vi "Display Info.vi"(7 "Layout ref":refnum<vi>, 8 "error in (no error)":errorcluster, 9 "Modify (F) /Add [T]":bool, 10 "Names in use":string[](array[string]), 11 "Advanced_DMD in":refnum<class "Advanced_DMD.lvclass">) -> (0 "error out":errorcluster, 1 "Names in use out":string[](array[string]), 2 "Changes Made?":bool, 3 "Advanced_DMD out":refnum<class "Advanced_DMD.lvclass">)   [LabVIEW 2013, in "Advanced_DMD.lvclass"]
uses:
  Advanced_DMD.lvclass
  TypeDefs/ColumnAppearCluster.ctl
  Advanced_DMD.lvclass/Advanced_DMD.ctl
  ColumnVIs/Column/Column.lvclass
panel:
  in  "Mode Appearance":T1={"Column Name"="Num Images", "Width"=30, "Bkgd"=[16448250], "Text"=[0]}
  in  "Image Cluster":T2
  in  "Argument Column Appearance":T1={"Column Name"="Column_0", "Width"=30, "Bkgd"=[16448250], "Text"=[0]}
  in  "Program Mode Appearance":T1={"Column Name"="Program Mode", "Width"=30, "Bkgd"=[16448250], "Text"=[0]}
  in  "Display Mode Appearance":T1={"Column Name"="Disp Mode", "Width"=30, "Bkgd"=[16448250], "Text"=[0]}
  in  "Device Description":string
  in  "Hardware Settings":T3={"IP Address"="172.16.1.100", "Image Root Path"=path "C:/Users/Lab/Google Drive/Sr/ToOrganize/Strontium Experiment/DLP3000 codes/Matlab codes/Sr_Matlab", "Port"=21845} {"Port" format="%x"}
  in  "Name":string
  in  "Done":bool
  in  "Cancel":bool
  # "Use IP addresses in: \n172.16.0.0 to 172.16.255.255\nor\n192.168.0.0 to 192.168.255.255\ncurrent setting: 172.16.1.100\n\nNote: Most DMDs default to\n192.168.1.100\n\nIf another IP is needed it must be \nset with the DMD software."
  # "This VI just sets the wiring structure.\nOpen a child override version instead!"
  # "Always use Port 0x5555\nPort Field is in Hexadecimal"
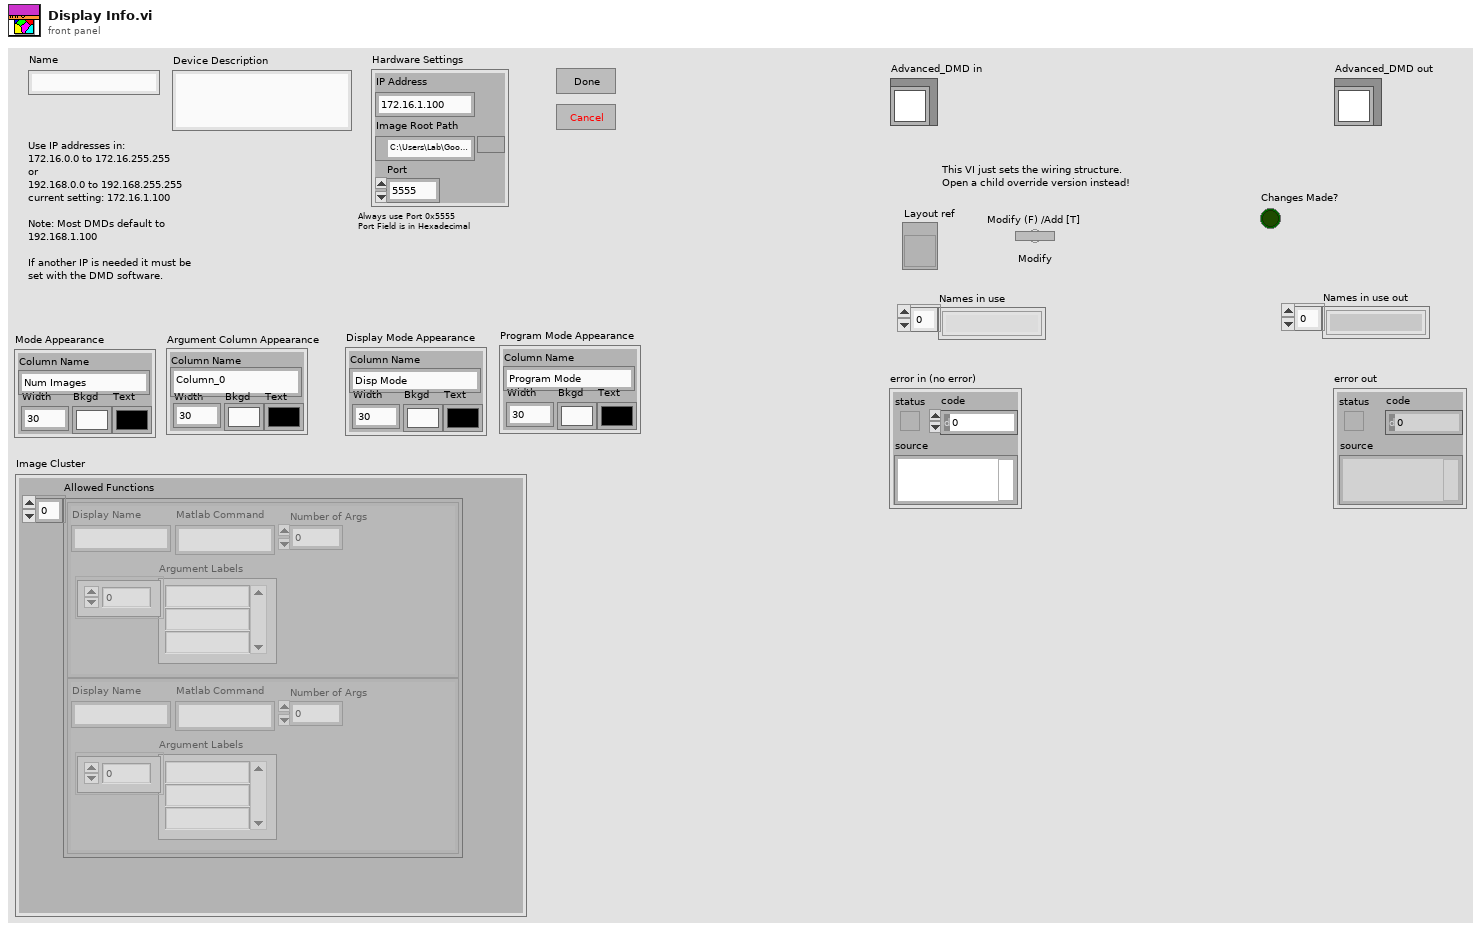
[diagram p1: front panel]
types:
  T1 = typedef "ColumnAppearCluster.ctl" = cluster{"Column Name":string, "Width":u32, "Bkgd":u32[], "Text":u32[]}
  T2 = cluster{"Allowed Functions":cluster{"Display Name":string, "Matlab Command":string, "Number of Args":u8, "Argument Labels":string[]}[]}
  T3 = cluster{"IP Address":string, "Image Root Path":path, "Port":u16}
  T4 = cluster{"Display Name":string, "Matlab Command":string, "Number of Args":u8, "Argument Labels":string[]}[]
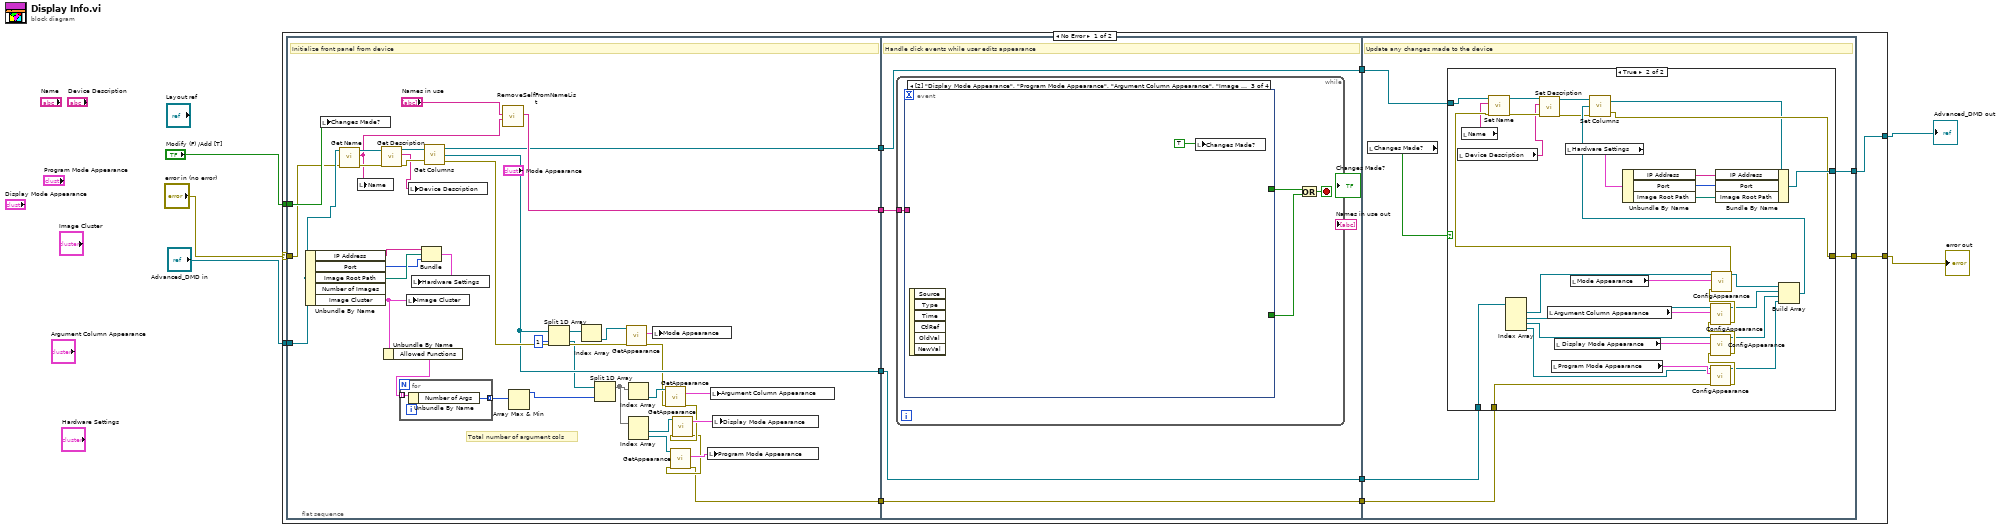
[diagram p0: block diagram]
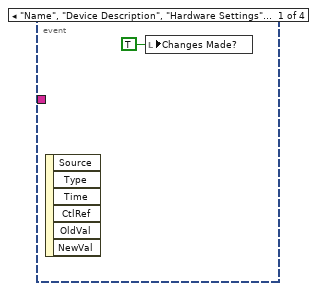
[diagram p2: hidden frame]
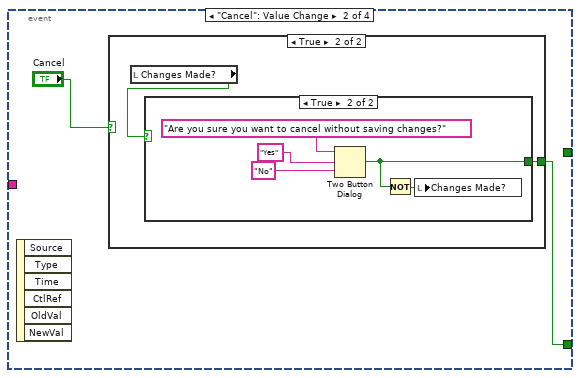
[diagram p3: hidden frame]
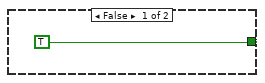
[diagram p5: hidden frame]
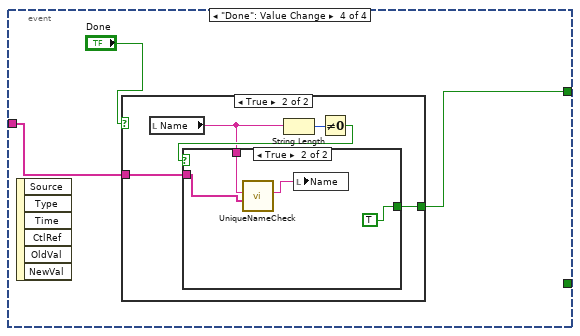
[diagram p6: hidden frame]
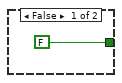
[diagram p7: hidden frame]
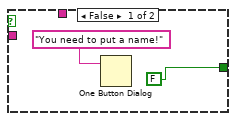
[diagram p8: hidden frame]
diagram:
  n1 = case shown="No Error" "error in (no error)" {
    selector: "error in (no error)" -> [w15 w136]
    tunnel: [w7 w136] -> w1
    tunnel: [w6 w135] -> w2
    tunnel: "Advanced_DMD in" -> [w16 w135]
    tunnel: "Modify (F) /Add [T]" -> [w17 _]
    frame No Error {
      n2 = flat-sequence {
        tunnel: w17 -> [w55]
        tunnel: w16 -> [w53]
        tunnel: w15 -> [w51]
        tunnel: [w43] -> w14
        tunnel: [w42] -> w13
        tunnel: [w35] -> w11
        tunnel: [w19] -> w9
        tunnel: w14 -> [w61]
        tunnel: w13 -> [w60]
        tunnel: [w60] -> w12
        tunnel: w11 -> [w59]
        tunnel: [w59] -> w10
        tunnel: w9 -> [w58]
        tunnel: [w58] -> w8
        tunnel: w12 -> [w99]
        tunnel: w10 -> [w98]
        tunnel: w8 -> [w97]
        tunnel: [w95] -> w7
        tunnel: [w94] -> w6
        frame #0 {
          # "Total number of argument cols"
          # "Initialize front panel from device"
          n3 = Unbundle By Name(w53) -> ("IP Address"=w54:string, "Port"=w40:u16, "Image Root Path"=w41:path, "Image Cluster"=w18:T2)  [unwired: 1 out]
          n4 = local write "Changes Made?"(w55) -> ()
          n5 = call-dynamic "Get Name.vi"("error in (no error)"=w51, "Device in"=w53) -> ("error out"=w50:errorcluster, "Name"=w47:string, "Device out"=w52:refnum<class "Advanced_DMD.lvclass">)  [unwired: 7 in]
          n6 = local write "Name"(w47) -> ()
          n7 = call-dynamic "Get Description.vi"("error in (no error)"=w50, "Device in"=w52) -> ("error out"=w48:errorcluster, "Device Description"=w46:string, "Device out"=w49:refnum<class "Advanced_DMD.lvclass">)  [unwired: 7 in]
          n8 = Unbundle By Name(w18) -> ("Allowed Functions"=w37:T4)
          n9 = for {
            tunnel: w37 -> [w57] mode=indexing
            tunnel: [w56] -> w36 mode=indexing
            n10 = Unbundle By Name(w57) -> ("Number of Args"=w56:u8)
          }
          n11 = local write "Image Cluster"(w18) -> ()
          n12 = local write "Device Description"(w46) -> ()
          n13 = Bundle("IP Address"=w54, "Image Root Path"=w41, "Port"=w40) -> (w39:T3)  [unwired: 1 in]
          n14 = local write "Hardware Settings"(w39) -> ()
          n15 = call-dynamic "Get Columns.vi"("Device in"=w49, "error in (no error)"=w48) -> ("Device out"=w42:refnum<class "Advanced_DMD.lvclass">, "Columns"=w35:refnum<class "Column.lvclass">[], "error out"=w45:errorcluster)
          n16 = call "RemoveSelfFromNameList.vi"("self Name"=w47, "Names in use"="Names in use") -> ("Reserved Names"=w43:string[])  [unwired: 9 in]
          n17 = Array Max & Min(array=w36) -> (max value=w31:u8)  [unwired: 3 out]
          n18 = Split 1D Array(array=w35, index=1) -> (first subarray=w33:refnum<class "Column.lvclass">[], second subarray=w30:refnum<class "Column.lvclass">[])
          n19 = Index Array(array=w33) -> (element=w32:refnum<class "Column.lvclass">)  [unwired: 1 in]
          n20 = Split 1D Array(array=w30, index=w31) -> (first subarray=w27:refnum<class "Column.lvclass">[])  [unwired: 1 out]
          n21 = call "GetAppearance.vi"("error in (no error)"=w45, "Column in"=w32) -> ("error out"=w22:errorcluster, "Column Appearance"=w44:T1)  [unwired: 7 in, 1 out]
          n22 = Index Array(array=w27) -> (element=w29:refnum<class "Column.lvclass">)  [unwired: 1 in]
          n23 = Index Array(array=w27) -> (element #1=w26:refnum<class "Column.lvclass">, element #2=w25:refnum<class "Column.lvclass">)  [unwired: 2 in]
          n24 = local write "Mode Appearance"(w44) -> ()
          n25 = call "GetAppearance.vi"("error in (no error)"=w22, "Column in"=w29) -> ("error out"=w21:errorcluster, "Column Appearance"=w28:T1)  [unwired: 7 in, 1 out]
          n26 = call "GetAppearance.vi"("error in (no error)"=w21, "Column in"=w26) -> ("error out"=w20:errorcluster, "Column Appearance"=w24:T1)  [unwired: 7 in, 1 out]
          n27 = call "GetAppearance.vi"("error in (no error)"=w20, "Column in"=w25) -> ("error out"=w19:errorcluster, "Column Appearance"=w23:T1)  [unwired: 7 in, 1 out]
          n28 = local write "Program Mode Appearance"(w23) -> ()
          n29 = local write "Argument Column Appearance"(w28) -> ()
          n30 = local write "Display Mode Appearance"(w24) -> ()
        }
        frame #1 {
          # "Handle click events while user edits appearance"
          n31 = while {
            tunnel: w61 -> [w62]
            stop <- w65 stop-if-true
            n32 = event shown="[2] \"Display Mode Appearance\", \"Program Mode Appearance\", \"Argument Column Appearance\", \"Image Cluster\", \"Mode Appearance\": Value Change" {
              selector: _ -> [_ _ _ _]
              dyn-events: _ -> [_ _ _ _]
              timeout: _ -> [_ _ _ _]
              tunnel: [_ w68 _ _] -> w64
              tunnel: [_ _ _ w81] -> w63
              tunnel: w62 -> [_ _ _ w80]
              event "Name", "Device Description", "Hardware Settings": Value Change {
                n33 = event-data() -> ()  [unwired: 1 in, 6 out]
                n34 = local write "Changes Made?"(TRUE ("Changes Made?")) -> ()
              }
              event "Cancel": Value Change {
                n35 = event-data() -> ()  [unwired: 1 in, 6 out]
                n36 = case shown="True" "Cancel" {
                  selector: "Cancel" -> [w69 _]
                  tunnel: [w69 w71] -> w68
                  frame False {
                  }
                  frame True {
                    n37 = local read "Changes Made?"() -> (w70:bool)
                    n38 = case shown="True" w70 {
                      tunnel: [TRUE w74] -> w71
                      frame False {
                      }
                      frame True {
                        n39 = Two Button Dialog(message="Are you sure you want to cancel without saving changes?", 1:"No", 2:"Yes") -> (T button?=w74:bool)
                        n40 = Not(x=w74) -> (.not. x?=w73:bool)
                        n41 = local write "Changes Made?"(w73) -> ()
                      }
                    }
                  }
                }
              }
              event "Image Cluster": Value Change {
                n42 = event-data() -> ()  [unwired: 1 in, 6 out]
                n43 = local write "Changes Made?"(TRUE) -> ()
              }
              event "Done": Value Change {
                n44 = event-data() -> ()  [unwired: 1 in, 6 out]
                n45 = case shown="True" "Done" {
                  tunnel: [FALSE w85] -> w81
                  tunnel: w80 -> [_ w84]
                  frame False {
                  }
                  frame True {
                    n46 = local read "Name"() -> (w83:string)
                    n47 = String Length(string=w83) -> (length=w87:i32)
                    n48 = Not Equal To 0?(x=w87) -> (x != 0?=w86:bool)
                    n49 = case shown="True" w86 {
                      tunnel: [FALSE TRUE] -> w85
                      tunnel: w84 -> [_ w92]
                      tunnel: w83 -> [_ w91]
                      frame False {
                        n50 = One Button Dialog(message="You need to put a name!") -> ()  [unwired: 1 in, 1 out]
                      }
                      frame True {
                        n51 = call "UniqueNameCheck.vi"("Names in use"=w92, "Device Name"=w91) -> ("Unique name"=w90:string)  [unwired: 8 in, 1 out]
                        n52 = local write "Name"(w90) -> ()
                      }
                    }
                  }
                }
              }
            }
            n53 = Or(x=w63, y=w64) -> (x .or. y?=w65:bool)
          }
        }
        frame #2 {
          # "Update any changes made to the device"
          n54 = local read "Changes Made?"() -> (w96:bool)
          n55 = case shown="True" w96 {
            tunnel: w99 -> [w101 w134]
            tunnel: w98 -> [_ w132]
            tunnel: w97 -> [w100 w109]
            tunnel: [w100 w111] -> w95
            tunnel: [w101 w114] -> w94
            frame False {
            }
            frame True {
              n56 = local read "Device Description"() -> (w102:string)
              n57 = local read "Name"() -> (w103:string)
              n58 = Index Array(array=w132) -> (element #1=w131:refnum<class "Column.lvclass">, element #2=w130:refnum<class "Column.lvclass">, element #3=w129:refnum<class "Column.lvclass">, element #4=w106:refnum<class "Column.lvclass">)  [unwired: 4 in]
              n59 = local read "Argument Column Appearance"() -> (w123:T1)
              n60 = local read "Program Mode Appearance"() -> (w107:T1)
              n61 = local read "Display Mode Appearance"() -> (w122:T1)
              n62 = local read "Hardware Settings"() -> (w104:T3)
              n63 = local read "Mode Appearance"() -> (w124:T1)
              n64 = Unbundle By Name(w104) -> ("IP Address"=w115:string, "Port"=w113:u16, "Image Root Path"=w112:path)
              n65 = call "ConfigAppearance.vi"("error in (no error)"=w109, "Column Appearance"=w107, "Column in"=w106) -> ("error out"=w108:errorcluster, "Column out"=w105:refnum<class "Column.lvclass">)  [unwired: 7 in]
              n66 = call "ConfigAppearance.vi"("error in (no error)"=w108, "Column Appearance"=w122, "Column in"=w129) -> ("error out"=w128:errorcluster, "Column out"=w119:refnum<class "Column.lvclass">)  [unwired: 7 in]
              n67 = call "ConfigAppearance.vi"("error in (no error)"=w128, "Column Appearance"=w123, "Column in"=w130) -> ("error out"=w127:errorcluster, "Column out"=w120:refnum<class "Column.lvclass">)  [unwired: 7 in]
              n68 = call "ConfigAppearance.vi"("error in (no error)"=w127, "Column Appearance"=w124, "Column in"=w131) -> ("error out"=w126:errorcluster, "Column out"=w121:refnum<class "Column.lvclass">)  [unwired: 7 in]
              n69 = call-dynamic "Set Name.vi"("error in (no error)"=w126, "Name"=w103, "Device in"=w134) -> ("error out"=w125:errorcluster, "Device out"=w133:refnum<class "Advanced_DMD.lvclass">)  [unwired: 7 in]
              n70 = call-dynamic "Set Description.vi"("error in (no error)"=w125, "Device Description"=w102, "Device in"=w133) -> ("error out"=w116:errorcluster, "Device out"=w117:refnum<class "Advanced_DMD.lvclass">)  [unwired: 7 in]
              n71 = Build Array(w121, w120, w119, w105) -> (w118:refnum<class "Column.lvclass">[])
              n72 = call-dynamic "Set Columns.vi"("error in (no error)"=w116, "Columns"=w118, "Device in"=w117) -> ("error out"=w111:errorcluster, "Device out"=w110:refnum<class "Advanced_DMD.lvclass">)  [unwired: 1 in]
              n73 = Bundle By Name(cluster=w110, "IP Address"=w115, "Port"=w113, "Image Root Path"=w112) -> (w114:refnum<class "Advanced_DMD.lvclass">)
            }
          }
        }
      }
    }
    frame Error {
    }
  }
  "error out" <- w1
  "Advanced_DMD out" <- w2
